vi "Read Waveform from TDMS.vi"() -> ()   [LabVIEW 2021, in "PMIC Common.lvlib"]
uses:
  PMIC Common.lvlib
panel:
  in  "Group Names":string[](array[string])
  in  "TDMS File Path":path=path "C:/Users/NIJ ASE/Desktop/results/Load Transient Response Vin_12.000 Iout1_2.000 Iout2_3.000.tdms"
  out "XY Graph":cluster{"time":dbl[], "waveform":dbl[]}[](graph)
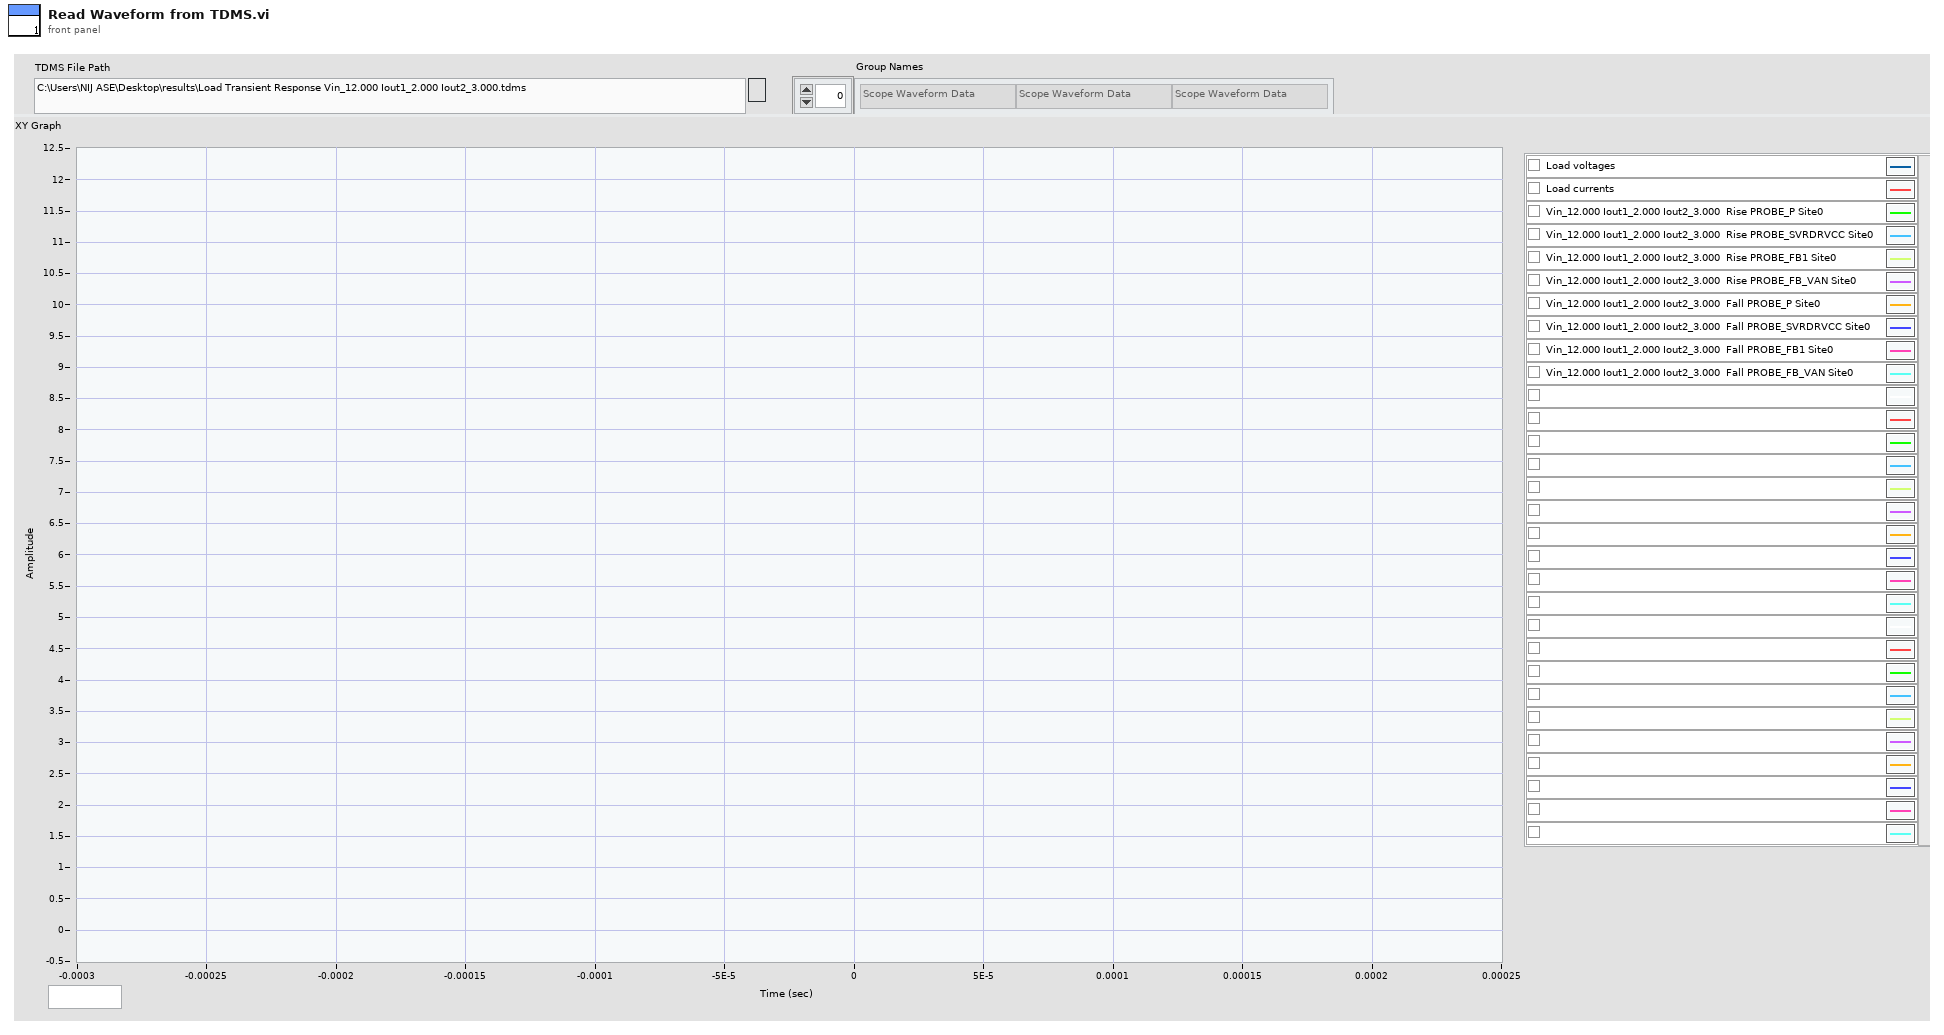
[diagram p1: front panel]
types:
  T1 = enum16{"open", "open or create", "create or replace", "create", "open (read-only)"}
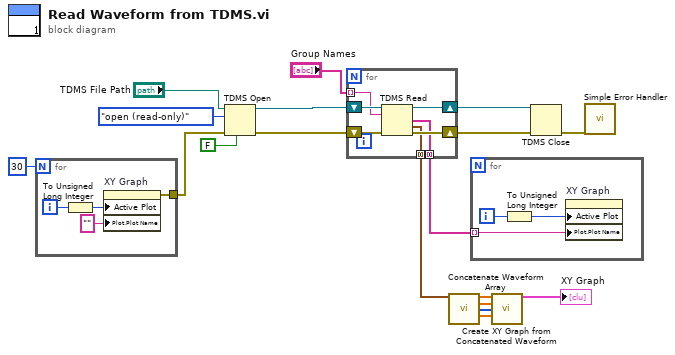
[diagram p0: block diagram]
diagram:
  n1 = for {
    N: 30 -> [_]
    tunnel: [w19] -> w7
    i -> [w22]
    n2 = To Unsigned Long Integer(number=w22) -> (unsigned 32bit integer=w21:u32)
    n3 = property on="XY Graph" class="XYGraph (strict)"("Active Plot"=w21, "Plot.Plot Name"="") -> (error out=w19:errorcluster)  [unwired: 2 in, 1 out]
  }
  n4 = TDMS Open(6:FALSE ("disable buffering? (T)"), 8:w7, 10:T1."open (read-only)" ("operation (0:open)"), 11:"TDMS File Path") -> (0:w15:errorcluster, 3:w16:refnum<k34>)  [unwired: 3 in]
  n5 = for {
    tunnel: [w25] -> w10 mode=concatenating
    tunnel: [w24] -> w2 mode=concatenating
    shift-right: [w27] -> w12
    shift-left: w16 -> [w29]
    shift-right: [w26] -> w11
    shift-left: w15 -> [w28]
    tunnel: "Group Names" -> [w23] mode=indexing
    n6 = TDMS Read(0:w29, 5:w23, 11:w28) -> (4:w27:refnum<k34>, 8:w25:string[], 10:w24:waveform(dbl)[], 15:w26:errorcluster)  [unwired: 5 in, 2 out]
  }
  n7 = call "Concatenate Waveform Array.vi"("waveform array"=w2) -> ("waveform t0 array"=w6:dbl[], "waveform dt array"=w5:dbl[], "waveform length array"=w4:i32[], "concatenated waveform Y"=w3:dbl[])  [unwired: 11 in]
  n8 = for {
    tunnel: w10 -> [w30] mode=indexing
    i -> [w32]
    n9 = To Unsigned Long Integer(number=w32) -> (unsigned 32bit integer=w31:u32)
    n10 = property on="XY Graph" class="XYGraph (strict)"("Active Plot"=w31, "Plot.Plot Name"=w30) -> ()  [unwired: 2 in, 2 out]
  }
  n11 = call "Create XY Graph from Concatenated Waveform.vi"("waveform t0 array"=w6, "waveform dt array"=w5, "waveform length array"=w4, "concatenated waveform Y"=w3) -> ("XY Graph Array"=→"XY Graph":cluster{"time":dbl[], "waveform":dbl[]}[])  [unwired: 11 in]
  n12 = TDMS Close(8:w11, 11:w12) -> (0:w13:errorcluster)  [unwired: 1 out]
  n13 = call <vilib>:"Simple Error Handler.vi"("error in (no error)"=w13) -> ()  [unwired: 4 in, 5 out]
